vi "声发射_幅值.vi"(10 "波峰位置":dbl[](array[numeric]), 11 "数据":dbl[](array[numeric])) -> (3 "幅值":dbl)   [LabVIEW 2014]
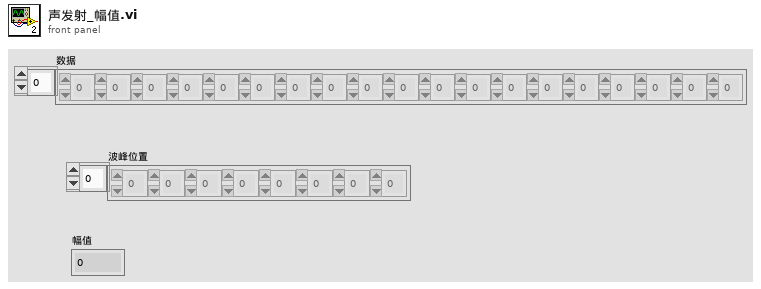
[diagram p1: front panel]
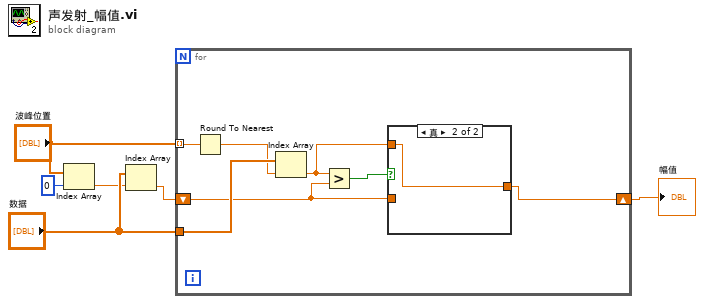
[diagram p0: block diagram]
diagram:
  n1 = Index Array(array="波峰位置", index=0 ("索引")) -> (element=w2:dbl)
  n2 = Index Array(array="数据", index=w2) -> (element=w1:dbl)
  n3 = for {
    tunnel: "波峰位置" -> [w13] mode=indexing
    shift-right: [w9] -> w4
    shift-left: w1 -> [w7]
    tunnel: "数据" -> [w12]
    n4 = Round To Nearest(number=w13) -> (nearest integer value=w10:dbl)
    n5 = Index Array(array=w12, index=w10) -> (element=w8:dbl)
    n6 = Greater?(x=w8, y=w7) -> (0:w11:bool)
    n7 = case shown="真" w11 {
      tunnel: [w14 w15] -> w9
      tunnel: w8 -> [_ w15]
      tunnel: w7 -> [w14 _]
      frame False {
      }
      frame True {
      }
    }
  }
  "幅值" <- w4
